vi "Create Platform Steering Frame.vi"(8 "error in (no error)":errorcluster) -> (0 "error out":errorcluster, 3 "KUKA youBot steering frame out":refnum<class "NI_Robotics_Mecanum Steering Frame.lvclass">)   [LabVIEW 2017, in "NI_Robotics_KUKA youBot Host.lvlib" / "NI_Robotics_KUKA youBot Platform.lvclass"]
doc: "Creates a steering frame based on the KUKA youBot mobile platform."
uses:
  <vilib>/robotics/KUKA youBot/Basic Device/Mobile Platform/NI_Robotics_KUKA youBot Platform.lvclass
  <vilib>/robotics/Steering/Mecanum Steering Frame/NI_Robotics_Mecanum Steering Frame.lvclass
  <vilib>/robotics/Steering/Wheel/Wheel Parameters.ctl
  <vilib>/robotics/Steering/Wheel/Rotation Direction.ctl
  <vilib>/robotics/Steering/Mecanum Wheel/Roller Orientation.ctl
  <vilib>/robotics/Steering/Mecanum Steering Frame/Create Mecanum Steering Frame.vi
  <vilib>/robotics/Steering/Mecanum Wheel/Create Mecanum Wheel.vi
  <vilib>/robotics/Steering/Wheel/NI_Robotics_Wheel.lvclass
  <vilib>/robotics/Steering/Mecanum Wheel/NI_Robotics_Mecanum Wheel.lvclass
  <vilib>/robotics/Steering/Steering Frame/NI_Robotics_Steering Frame.lvclass
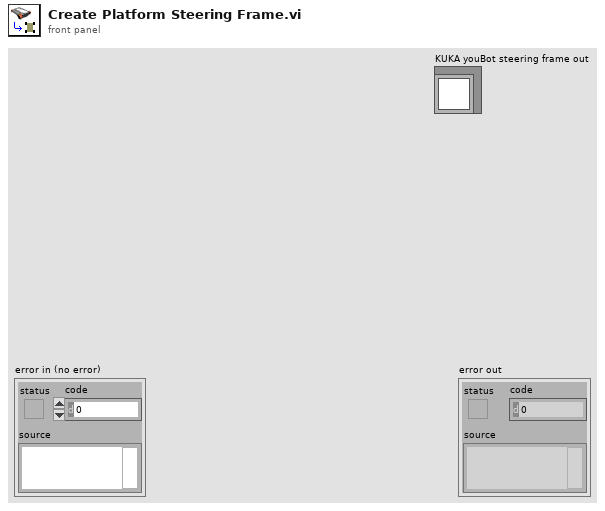
[diagram p1: front panel]
types:
  T1 = typedef "NI_Robotics_Wheel.lvclass/Wheel Parameters.ctl" = cluster{"wheel radius":dbl, "gear ratio":dbl, "forward rotation direction":T2}
  T2 = typedef "NI_Robotics_Wheel.lvclass/Rotation Direction.ctl" = u16
  T3 = typedef "NI_Robotics_Mecanum Wheel.lvclass/Roller Orientation.ctl" = u16
  T4 = cluster{"[0]":refnum<class "NI_Robotics_Mecanum Wheel.lvclass">, "[1]":refnum<class "NI_Robotics_Mecanum Wheel.lvclass">, "[2]":refnum<class "NI_Robotics_Mecanum Wheel.lvclass">, "[3]":refnum<class "NI_Robotics_Mecanum Wheel.lvclass">}
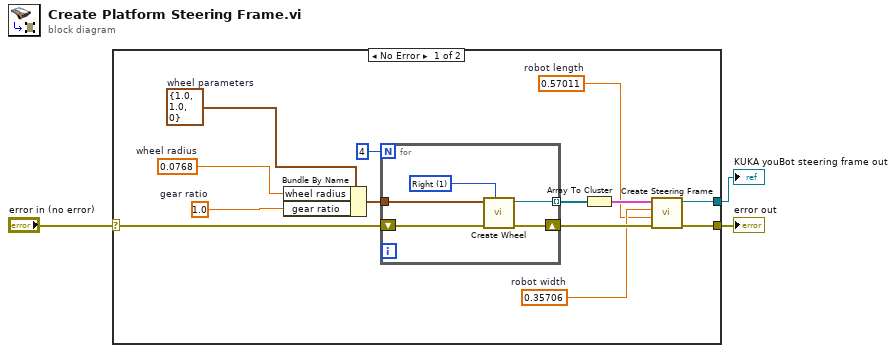
[diagram p0: block diagram]
diagram:
  n1 = case shown="No Error" "error in (no error)" {
    selector: "error in (no error)" -> [w10 w22]
    tunnel: [w9 w22] -> w1
    tunnel: [w8 _] -> w3
    frame No Error {
      w5 = 0.35706  # robot width
      w4 = 0.57011  # robot length
      w6 = 1.0  # gear ratio
      w7 = 0.0768  # wheel radius
      w15 = T1 {"wheel radius"=1.0, "gear ratio"=1.0, "forward rotation direction"=0}  # wheel parameters
      n2 = Bundle By Name(cluster=w15, "wheel radius"=w7, "gear ratio"=w6) -> (w16:T1)
      n3 = for {
        N: 4 -> [_]
        shift-right: [w20] -> w12
        shift-left: w10 -> [w21]
        tunnel: [w19] -> w14 mode=indexing
        tunnel: w16 -> [w18]
        w17 = T3 1 items=["Left", "Right"] ("roller orientation")
        n4 = call-poly <vilib>:"Create Wheel.vi"("roller orientation"=w17, "error in (no error)"=w21, "wheel parameters"=w18) -> ("error out"=w20:errorcluster, "mecanum wheel out"=w19:refnum<class "NI_Robotics_Mecanum Wheel.lvclass">)  [unwired: 7 in]
      }
      n5 = Array To Cluster(array=w14) -> (cluster=w13:T4)
      n6 = call-poly <vilib>:"Create Steering Frame.vi"("error in (no error)"=w12, "wheel separation length"=w4, "wheel separation width"=w5, "wheels"=w13) -> ("error out"=w9:errorcluster, "mecanum steering frame out"=w8:refnum<class "NI_Robotics_Mecanum Steering Frame.lvclass">)  [unwired: 6 in]
    }
    frame Error {
    }
  }
  "error out" <- w1
  "KUKA youBot steering frame out" <- w3
